vi "Read Alias.vi"(8 "error in (no error)":errorcluster, 11 "DeployResource in":refnum<class "Resource.lvclass">) -> (0 "error out":errorcluster, 2 "Alias":string, 3 "DeployResource out":refnum<class "Resource.lvclass">)   [LabVIEW 2020, in "PicoG-Core.lvlib" / "Resource.lvclass"]
uses:
  Resource.lvclass
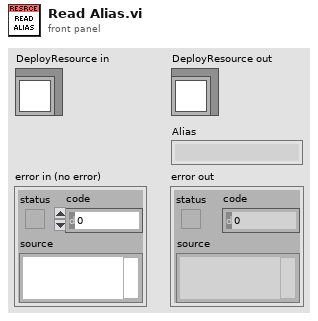
[diagram p1: front panel]
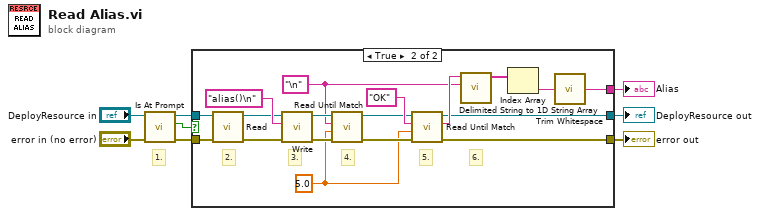
[diagram p0: block diagram]
diagram:
  # "1."
  n1 = call-dynamic "Is At Prompt.vi"("error in (no error)"="error in (no error)", "DeployResource in"="DeployResource in") -> ("error out"=w4:errorcluster, "At Prompt?"=w6:bool, "DeployResource out"=w5:refnum<class "Resource.lvclass">)  [unwired: 6 in, 1 out]
  n2 = case shown="True" w6 {
    tunnel: w5 -> [w10 w27]
    tunnel: w4 -> [w9 w26]
    tunnel: [w10 w20] -> w3
    tunnel: [w9 w19] -> w2
    tunnel: [_ w11] -> w1
    frame False {
      # "#ERROR"
    }
    frame True {
      w12 = 5.0 ("Timeout S (0)")
      w13 = "\n" ("Data")
      # "6."
      # "5."
      # "4."
      # "3."
      # "2."
      n3 = call "Read.vi"("error in (no error)"=w26, "DeployResource in"=w27) -> ("error out"=w24:errorcluster, "DeployResource out"=w25:refnum<class "Resource.lvclass">)  [unwired: 6 in, 2 out]
      n4 = call "Write.vi"("error in (no error)"=w24, "Data"="alias()\n", "DeployResource in"=w25) -> ("error out"=w16:errorcluster, "DeployResource out"=w17:refnum<class "Resource.lvclass">)  [unwired: 6 in, 1 out]
      n5 = call "Read Until Match.vi"("error in (no error)"=w16, "Timeout S (0)"=w12, "Match String"=w13, "DeployResource in"=w17) -> ("error out"=w14:errorcluster, "DeployResource out"=w15:refnum<class "Resource.lvclass">)  [unwired: 4 in, 2 out]
      n6 = call "Read Until Match.vi"("error in (no error)"=w14, "Timeout S (0)"=w12, "Match String"="OK" ("Data"), "DeployResource in"=w15) -> ("error out"=w19:errorcluster, "Data"=w23:string, "DeployResource out"=w20:refnum<class "Resource.lvclass">)  [unwired: 4 in, 1 out]
      n7 = call <vilib>:"Delimited String to 1D String Array.vi"("delimiter"=w13, "delimited string"=w23) -> ("string array"=w22:string[])  [unwired: 9 in]
      n8 = Index Array(array=w22) -> (element=w21:string)  [unwired: 1 in]
      n9 = call <vilib>:"Trim Whitespace.vi"("string"=w21) -> ("trimmed string"=w11:string)  [unwired: 1 in]
    }
  }
  "error out" <- w2
  "DeployResource out" <- w3
  "Alias" <- w1
